vi "Regresion_el_cal.vi"(10 "Angles in":T1) -> (1 "Offset":string, 2 "Slope":string, 3 "F-format string":string)   [LabVIEW 2018]
uses:
  SupportVIs/NI_AALPro.lvlib
  SupportVIs/NI_Gmath.lvlib
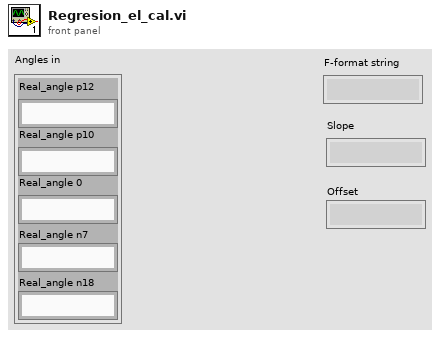
[diagram p1: front panel]
types:
  T1 = cluster{"Real_angle p12":string, "Real_angle p10":string, "Real_angle 0":string, "Real_angle n7":string, "Real_angle n18":string}
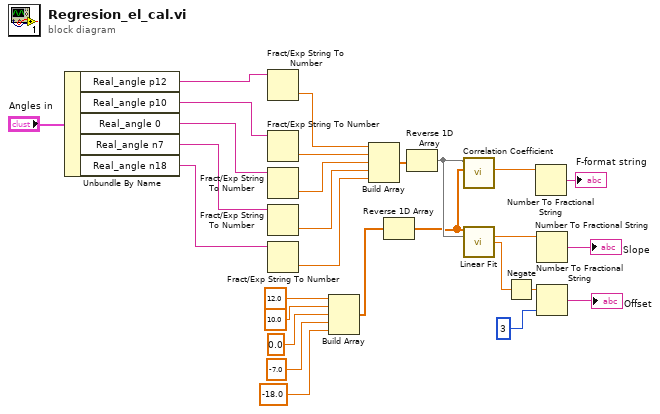
[diagram p0: block diagram]
diagram:
  n1 = Unbundle By Name("Angles in") -> ("Real_angle p12"=w14:string, "Real_angle p10"=w13:string, "Real_angle 0"=w12:string, "Real_angle n7"=w11:string, "Real_angle n18"=w10:string)
  n2 = Fract/Exp String To Number(string=w14) -> (number=w26:dbl)  [unwired: 3 in, 1 out]
  n3 = Fract/Exp String To Number(string=w13) -> (number=w25:dbl)  [unwired: 3 in, 1 out]
  n4 = Fract/Exp String To Number(string=w12) -> (number=w24:dbl)  [unwired: 3 in, 1 out]
  n5 = Fract/Exp String To Number(string=w11) -> (number=w23:dbl)  [unwired: 3 in, 1 out]
  n6 = Fract/Exp String To Number(string=w10) -> (number=w22:dbl)  [unwired: 3 in, 1 out]
  n7 = Build Array(12.0 ("element"), 10.0 ("element"), 0.0 ("element"), -7.0 ("element"), -18.0 ("element")) -> (w16:dbl[])
  n8 = Build Array(w26, w25, w24, w23, w22) -> (w8:dbl[])
  n9 = Reverse 1D Array(array=w16) -> (reversed array=w3:dbl[])
  n10 = Reverse 1D Array(array=w8) -> (reversed array=w4:dbl[])
  n11 = call "Correlation Coefficient.vi"("Y"=w3, "X"=w4) -> ("r^2"=w5:dbl)  [unwired: 8 in, 1 out]
  n12 = call "Linear Fit.vi"("Y"=w3, "X"=w4) -> ("slope"=w1:dbl, "intercept"=w9:dbl)  [unwired: 9 in, 3 out]
  n13 = Negate(x=w9) -> (-x=w7:dbl)
  n14 = Number To Fractional String(number=w5) -> (F-format string=→"F-format string":string)  [unwired: 3 in]
  n15 = Number To Fractional String(number=w1) -> (F-format string=→"Slope":string)  [unwired: 3 in]
  n16 = Number To Fractional String(number=w7, precision (6)=i16 3) -> (F-format string=→"Offset":string)  [unwired: 2 in]
